vi "FromRepo.vi"(8 "error in":errorcluster, 9 "from repo cluster":T2, 10 "repository in":refnum<class "NISE_CEF_Repository.lvclass">, 11 "node in":refnum<class "Initialization.lvclass">) -> (0 "error out":errorcluster, 2 "repository out":refnum<class "NISE_CEF_Repository.lvclass">, 3 "node":T1)   [LabVIEW 2015, in "Initialization.lvclass"]
doc: "Grabs information from the Repo and stores it in the nodes."
uses:
  Initialization.lvclass
  <vilib>/NI/Configuration Framework/Repository/NISE_CEF_Repository.lvclass
  <vilib>/NI/Configuration Framework/Node/FromRepoCluster.ctl
  <vilib>/NI/Configuration Framework/Node/NodeRef.ctl
  <vilib>/NI/Configuration Framework/Node/NISE_CEF_Node.lvclass
  CustomDeviceRepo/CustomDeviceRepo.lvclass
  CustomDeviceRepo/CustomDeviceRepo.lvclass/CustomDeviceRepo.ctl
  Initialization.lvclass/Initialization.ctl
  CustomDeviceRepo/Read Initialization VI Properties.vi
  Write Initialization VI Properties.vi
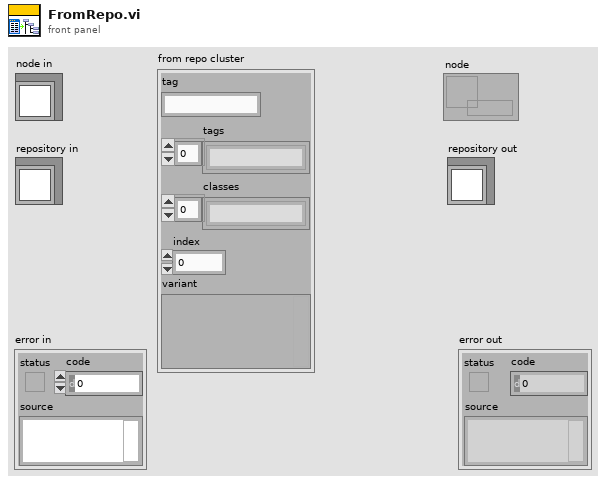
[diagram p1: front panel]
types:
  T1 = typedef "NISE_CEF_Node.lvclass/NodeRef.ctl" = refnum<data-value>
  T2 = typedef "NISE_CEF_Node.lvclass/FromRepoCluster.ctl" = cluster{"tag":string, "tags":string[], "classes":string[], "index":i32, "variant":variant}
  T3 = typedef "Initialization VI Properties.ctl" = cluster{"Execution":T4, "Path":T5, "Type":enum16{"Action", "VI"}, "Position":enum16{"centered", "mouse pointer"}}
  T4 = typedef "Execution Types.ctl" = enum16{"silent", "modal", "floating", "default"}
  T5 = typedef "Path Cluster.ctl" = cluster{"Path":path, "Path Type":enum16{"Absolute", "To Base", "To Common Doc Dir", "To Application Data Dir"}}
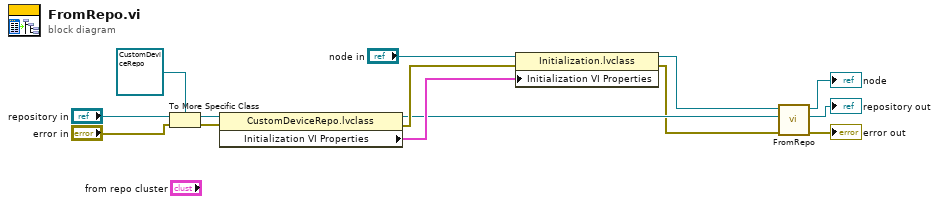
[diagram p0: block diagram]
diagram:
  n1 = To More Specific Class(target class=refnum<class "CustomDeviceRepo.lvclass"> refnum, reference="repository in", error in="error in") -> (specific class reference=w8:refnum<class "CustomDeviceRepo.lvclass">, error out=w7:errorcluster)
  n2 = property class="CustomDeviceRepo.lvclass"(reference=w8, error in=w7) -> (reference out=w2:refnum<class "CustomDeviceRepo.lvclass">, error out=w4:errorcluster, "Initialization VI Properties"=w5:T3)
  n3 = property class="Initialization.lvclass"(reference="node in", error in=w4, "Initialization VI Properties"=w5) -> (reference out=w3:refnum<class "Initialization.lvclass">, error out=w1:errorcluster)
  n4 = call-parent "FromRepo.vi"("error in"=w1, "repository in"=w2, "node in"=w3) -> ("error out"=→"error out":errorcluster, "repository out"=→"repository out":refnum<class "NISE_CEF_Repository.lvclass">, "node"=→"node":T1)  [unwired: 6 in]
